vi "getIVmode.vi"(8 "error in (no error)":errorcluster, 11 "Instrument.Lockin in":refnum<class "Instrument.Lockin.lvclass">) -> (0 "error out":errorcluster, 2 "IV mode":bool, 3 "Instrument.Lockin out":refnum<class "Instrument.Lockin.lvclass">)   [LabVIEW 2016, in "Instrument.Lockin.lvclass"]
doc: "API to get the results of lockin calculation.\n\nIf address=\"\", this API reads from localhost\nIf address is remote lockin, you need to add this computer to allowed whitelist on the lockin computer you are trying to access."
uses:
  Instrument.Lockin.lvclass
  Typedefs/Instrument.Lockin.Commands--Enum.ctl
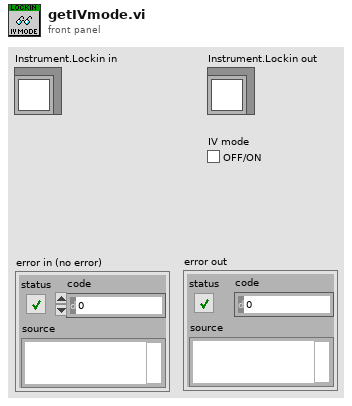
[diagram p1: front panel]
types:
  T1 = typedef "Instrument.Lockin.lvclass/Instrument.Lockin.Commands--Enum.ctl" = enum16{"setAO", "setAO_Amplitude", "setAO_DC", "setAO_Frequency", "setAO_Phase", "setAO_Function", "setAO_I+", "setREF", "setREF_Frequency", "setREF_Phase", "setIVmode", "Reset", "setSampling", "Trigger", "getAO", "getAI", "getResults", "getTrigger", "getIVmode", "getSampling", "getAOconfig", "getREFconfig", "setGain", "getGain", "setAutoSampling", "getAutoSampling", "setSweep", "getStatus", "getSweepResults", "startSweep", "stopSweep", "setAUX", "getAUX"}
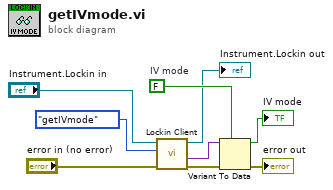
[diagram p0: block diagram]
diagram:
  w7 = FALSE  # IV mode
  n1 = call "Lockin Client.vi"("error in (no error)"="error in (no error)", "Command"=Instrument.Lockin.Commands--Enum."getIVmode", "Instrument.Lockin in"="Instrument.Lockin in") -> ("error out"=w5:errorcluster, "Data out"=w1:variant, "Instrument.Lockin out"=→"Instrument.Lockin out":refnum<class "Instrument.Lockin.lvclass">)  [unwired: 6 in]
  n2 = Variant To Data(error in=w5, type=w7, Variant=w1) -> (data=→"IV mode":bool, error out=→"error out":errorcluster)
